vi "PV Operating adjustment turbopump.vi"(8 "error in (no error)":errorcluster, 9 "Operating adjustment - Cluster":T1={"Parameter"=0, "Parameter\nread only<->describe"=FALSE, "off<->on"=TRUE, "Rotation speed set value\nin rot. speed setting\noperations [%]"=50.0, "Preset rotation Speed\nat Standby mode (%)"=66.0, "maximum power\nsetpoint [%]"=100, "Gas mode"=0} {"Gas mode" items=["heavy inert gases", "other gases", "helium"]; "maximum power\nsetpoint [%]" min=10 max=100 step=1; "Preset rotation Speed\nat Standby mode (%)" min=20.0 max=100.0 step=0.1 format="%.2f"; "Rotation speed set value\nin rot. speed setting\noperations [%]" min=20.0 max=100.0 step=0.1 format="%.2f"; "Parameter" items=[" Standby", " Pumping station", " Motor Turbopump", " Oper. mode TMP", " Gas mode", " Operating mode drive unit", " Rotation speed set value in rot. speed setting operations", " Set rotation speed TMP [Hz] (read only)", " Actual rotation speed TMP [Hz] (read only)", " Preset rotation Speed at Standby mode (%)", " Max. rotations speed ", " maximum power setpoint"]}, 10 "Adress of unit":u16=1 min=1 max=999 step=1, 11 "VISA session":refnum<visa-resource-name>) -> (0 "error out":errorcluster, 2 "response (data)":string, 3 "dup VISA session":refnum<visa-resource-name>)   [LabVIEW 2018, in "Pfeiffer Vacuum.lvlib"]
doc: "There are 12 parameters available, only one of which can be enabled at a time. \n\n0 - Stand by (default) (Para. 002)\n1 - Pumping station (Para. 010)\n2 - Motor Turbopump (Para. 023)\n3 - Oper. mode TMP (Para. 026)\n4 - Gas mode (Para. 027)\n5 - Operating mode drive unit (Para. 029)\n6 - Rotation speed set value in rot. speed setting operations (Para. 707)\n7 - Set rotation speed TMP [Hz] (read only) (Para. 308)\n8 - Actual rotation speed TMP [Hz] (read only) (Para. 309)\n9 - Preset rotation Speed at Standby mode (%) (Para. 717)\n10 - Max.rotation speed (Para.777)\n11 - maximum power setpoint (Para. 708)\n\nNote: The controls right of this one will set the appropriate values for the selected parameter. Any settings for an parameter that is not selected will be ignored. If a value is out of range, it will be changed to either the upper or the lower limit of the range."
uses:
  Pfeiffer Vacuum.lvlib
  PV Operating adjustment - Cluster.ctl
panel:
  # "Standby                                     :\n Pumping station                      :     \n Motor turbopump                    :\n Operations mode TMP           :\n Operating mode drive unit   :"
  # "<--------------\n  off\n  off\n  off\n  final rot. speed oper.       \n  max."
  # "----------->                 \non \non \non \nrot. speed setting \n reduced power consumpt."
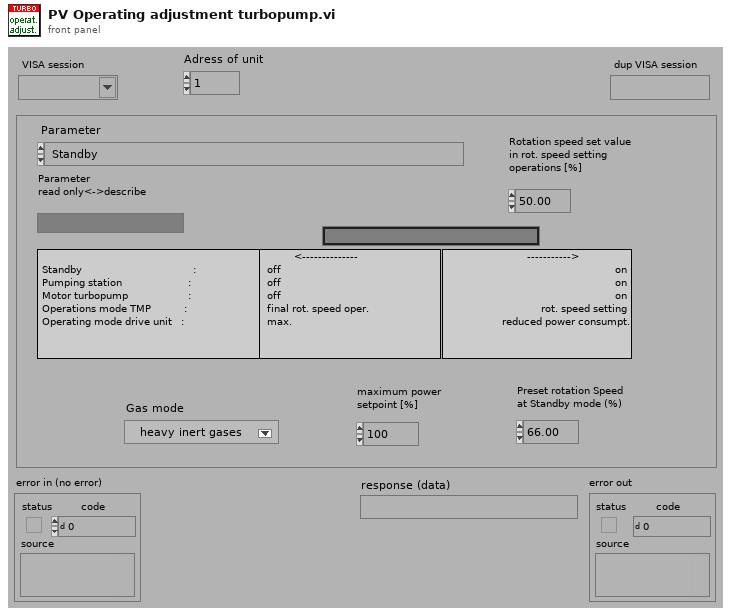
[diagram p1: front panel]
types:
  T1 = typedef "Pfeiffer Vacuum.lvlib/PV Operating adjustment - Cluster.ctl" = cluster{"Parameter":u16, "Parameter\nread only<->describe":bool, "off<->on":bool, "Rotation speed set value\nin rot. speed setting\noperations [%]":dbl, "Preset rotation Speed\nat Standby mode (%)":dbl, "maximum power\nsetpoint [%]":i32, "Gas mode":u16}
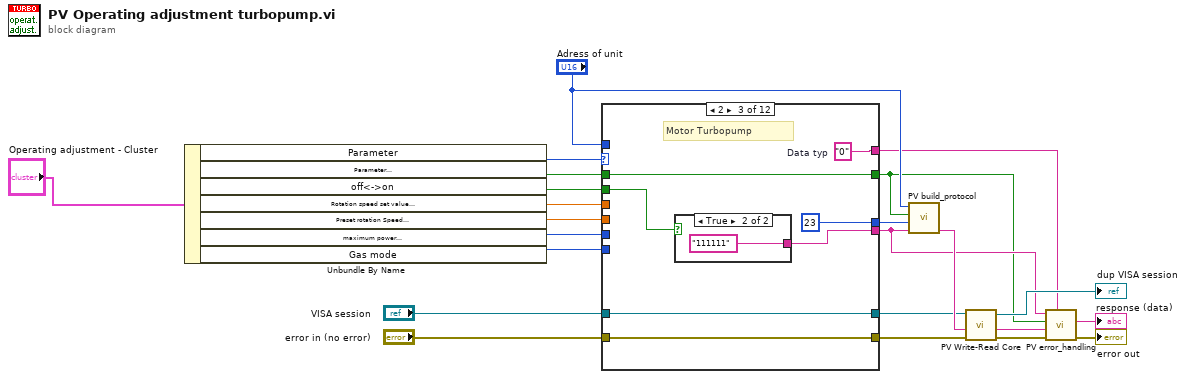
[diagram p0: block diagram]
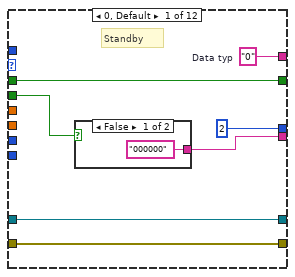
[diagram p2: hidden frame]
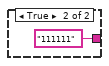
[diagram p3: hidden frame]
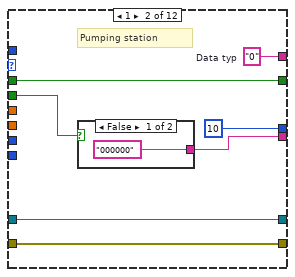
[diagram p4: hidden frame]
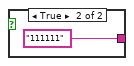
[diagram p5: hidden frame]
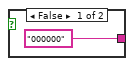
[diagram p6: hidden frame]
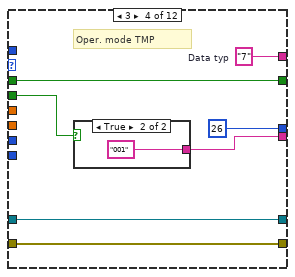
[diagram p7: hidden frame]
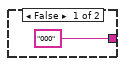
[diagram p8: hidden frame]
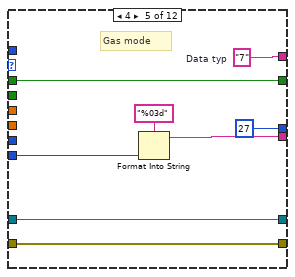
[diagram p9: hidden frame]
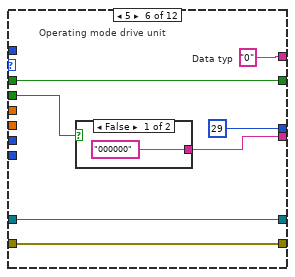
[diagram p10: hidden frame]
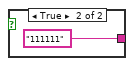
[diagram p11: hidden frame]
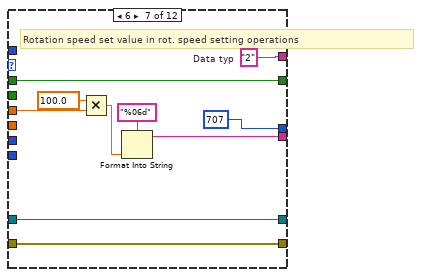
[diagram p12: hidden frame]
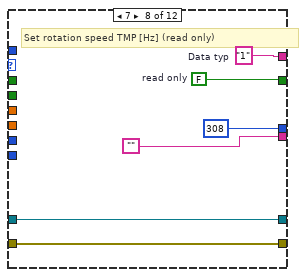
[diagram p13: hidden frame]
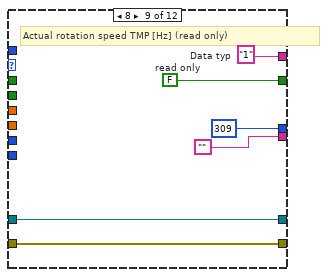
[diagram p14: hidden frame]
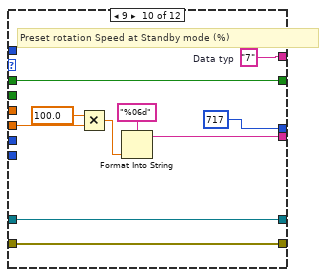
[diagram p15: hidden frame]
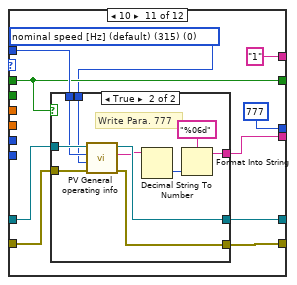
[diagram p16: hidden frame]
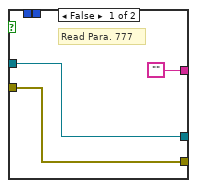
[diagram p17: hidden frame]
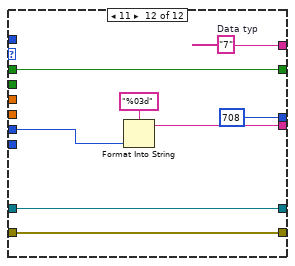
[diagram p18: hidden frame]
diagram:
  n1 = Unbundle By Name("Operating adjustment - Cluster") -> ("Parameter"=w22:u16, "Parameter\nread only<->describe"=w21:bool, "off<->on"=w20:bool, "Rotation speed set value\nin rot. speed setting\noperations [%]"=w19:dbl, "Preset rotation Speed\nat Standby mode (%)"=w18:dbl, "maximum power\nsetpoint [%]"=w3:i32, "Gas mode"=w1:u16)
  n2 = case shown="2" w22 {
    tunnel: [u16 2 ("Parameter-number") u16 10 ("Parameter-number") u16 23 ("Parameter-number") u16 26 ("Parameter-number") u16 27 ("Parameter-number") u16 29 ("Parameter-number") u16 707 ("Parameter-number") u16 308 ("Parameter-number") u16 309 ("Parameter-number") u16 717 ("Parameter-number") u16 777 ("Parameter-number") u16 708 ("Parameter-number")] -> w23
    tunnel: [w29 w38 w47 w56 w60 w73 w85 "" "" w107 w114 w132] -> w8
    tunnel: [w28 w37 w46 w55 w66 w72 w82 w91 w97 w105 w112 w135] -> w6
    tunnel: w21 -> [w28 w37 w46 w55 w66 w72 w82 _ _ w105 w112 w135]
    tunnel: w20 -> [w27 w36 w45 w54 _ w71 _ _ _ _ _ _]
    tunnel: w19 -> [_ _ _ _ _ _ w83 _ _ _ _ _]
    tunnel: [w26 w35 w44 w53 w65 w70 w79 w89 w95 w102 "1" ("Data typ") w137] -> w7
    tunnel: w18 -> [_ _ _ _ _ _ _ _ _ w101 _ _]
    tunnel: "VISA session" -> [w25 w34 w43 w52 w64 w69 w78 w88 w94 w100 w116 w139]
    tunnel: [w25 w34 w43 w52 w64 w69 w78 w88 w94 w100 w115 w139] -> w13
    tunnel: "Adress of unit" -> [_ _ _ _ _ _ _ _ _ _ w113 _]
    tunnel: "error in (no error)" -> [w24 w33 w42 w51 w63 w68 w77 w87 w93 w99 w111 w138]
    tunnel: [w24 w33 w42 w51 w63 w68 w77 w87 w93 w99 w110 w138] -> w12
    tunnel: w3 -> [_ _ _ _ _ _ _ _ _ _ _ w133]
    tunnel: w1 -> [_ _ _ _ w61 _ _ _ _ _ _ _]
    frame 0, Default {
      w26 = "0"  # Data typ
      # "Standby"
      n3 = case shown="False" w27 {
        tunnel: ["000000" ("Data") "111111" ("Data")] -> w29
        frame False {
        }
        frame True {
        }
      }
    }
    frame 1 {
      w35 = "0"  # Data typ
      # "Pumping station"
      n4 = case shown="False" w36 {
        tunnel: ["000000" ("Data") "111111" ("Data")] -> w38
        frame False {
        }
        frame True {
        }
      }
    }
    frame 2 {
      w44 = "0"  # Data typ
      # "Motor Turbopump"
      n5 = case shown="True" w45 {
        tunnel: ["000000" ("Data") "111111" ("Data")] -> w47
        frame False {
        }
        frame True {
        }
      }
    }
    frame 3 {
      w53 = "7"  # Data typ
      # "Oper. mode TMP"
      n6 = case shown="True" w54 {
        tunnel: ["000" ("Data") "001" ("Data")] -> w56
        frame False {
        }
        frame True {
        }
      }
    }
    frame 4 {
      w65 = "7"  # Data typ
      # "Gas mode"
      n7 = Format Into String(format string="%03d" ("Format-String"), w61) -> (resulting string=w60:string)  [unwired: 2 in, 1 out]
    }
    frame 5 {
      w70 = "0"  # Data typ
      # "Operating mode drive unit"
      n8 = case shown="False" w71 {
        tunnel: ["000000" ("Data") "111111" ("Data")] -> w73
        frame False {
        }
        frame True {
        }
      }
    }
    frame 6 {
      w79 = "2"  # Data typ
      # "Rotation speed set value in rot. speed setting operations"
      n9 = Multiply(x=100.0, y=w83) -> (x*y=w81:dbl)
      n10 = Format Into String(format string="%06d" ("Format-String"), w81) -> (resulting string=w85:string)  [unwired: 2 in, 1 out]
    }
    frame 7 {
      w89 = "1"  # Data typ
      w91 = FALSE  # read only
      # "Set rotation speed TMP [Hz] (read only)"
    }
    frame 8 {
      w95 = "1"  # Data typ
      w97 = FALSE  # read only
      # "Actual rotation speed TMP [Hz] (read only)"
    }
    frame 9 {
      w102 = "7"  # Data typ
      # "Preset rotation Speed at Standby mode (%)"
      n11 = Multiply(x=100.0, y=w101) -> (x*y=w104:dbl)
      n12 = Format Into String(format string="%06d" ("Format-String"), w104) -> (resulting string=w107:string)  [unwired: 2 in, 1 out]
    }
    frame 10 {
      w109 = u16 0 items=["nominal speed [Hz] (default) (315)", "intermediate circut current [A] (310)", "motor voltage [V] (313)", "actual power [W] (316)", "operating hours pump [h] (311)", "operating hours drive [h] (314)", "pump cycles (read only) (319)", "status oil sensor (read only) (301)", "speed switchpoint attained (read only) (302)", "overtemperature drive (read only) (304)", "overtemperature pump (read only) (305)", "target speed attained (read only) (306)", "pump accelerates (read only) (307) ", "controlled by remote (300)", "motor phase current [A] (317)", "acceleration / deceleration [rm/s] (336)", "hardware version controller (354)", "target speed (397)", "acutal speed (398)", "nominal speed (399)", "software version control unit (read only) (352)"] ("Parameter")
      n13 = case shown="True" w112 {
        tunnel: w116 -> [w121 w131]
        tunnel: [w121 w130] -> w115
        tunnel: ["" w124] -> w114
        tunnel: w113 -> [_ w129]
        tunnel: w111 -> [w119 w128]
        tunnel: w109 -> [_ w122]
        tunnel: [w119 w123] -> w110
        frame False {
          # "Read Para. 777"
        }
        frame True {
          # "Write Para. 777"
          n14 = call "PV General operating info.vi"("error in (no error)"=w128, "Parameter"=w122, "Adress of unit"=w129, "VISA session"=w131) -> ("error out"=w123:errorcluster, "response (data)"=w125:string, "dup VISA session"=w130:refnum<visa-resource-name>)  [unwired: 5 in]
          n15 = Decimal String To Number(string=w125) -> (number=w126:i32)  [unwired: 2 in, 1 out]
          n16 = Format Into String(format string="%06d" ("Format-String"), w126) -> (resulting string=w124:string)  [unwired: 2 in, 1 out]
        }
      }
    }
    frame 11 {
      w137 = "7"  # Data typ
      n17 = Format Into String(format string="%03d" ("Format-String"), w133) -> (resulting string=w132:string)  [unwired: 2 in, 1 out]
    }
  }
  n18 = call "PV build_protocol.vi"("Data"=w8, "Parameter-number"=w23, "parameter\nread<->describe"=w6, "Adress"="Adress of unit") -> ("output"=w14:string)  [unwired: 3 in]
  n19 = call "PV Write-Read Core.vi"("error in"=w12, "Write data in"=w14, "VISA session"=w13) -> ("error out"=w10:errorcluster, "response (data) out"=w11:string, "dup VISA session"=→"dup VISA session":refnum<visa-resource-name>)  [unwired: 2 in]
  n20 = call "PV error_handling.vi"("Data Typ in"=w7, "error in"=w10, "response (data) in"=w11, "Parameter\nread only<->describe"=w6, "data in"=w8) -> ("error out"=→"error out":errorcluster, "Data out"=→"response (data)":string)  [unwired: 4 in, 1 out]
